vi "Get All CEID Data.vi"(8 "error in (no error)":errorcluster) -> (0 "error out":errorcluster, 3 "CEID Data":T1[](array[typedef]))   [LabVIEW 2020, in "SECS Communication.lvlib" / "SECS Data Class.lvclass"]
uses:
  SECS Data Class.lvclass
  CEID Data.ctl
  SECS Data Class.lvclass/SECS Data Class.ctl
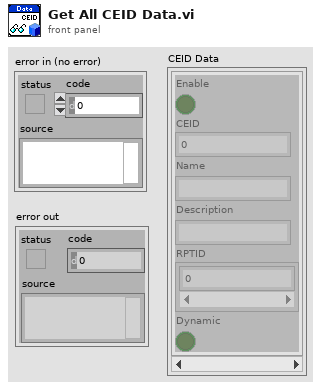
[diagram p1: front panel]
types:
  T1 = typedef "SECS Communication.lvlib/SECS Data Class.lvclass/CEID Data.ctl" = cluster{"Enable":bool, "CEID":u32, "Name":string, "Description":string, "RPTID":u32[], "Dynamic":bool}
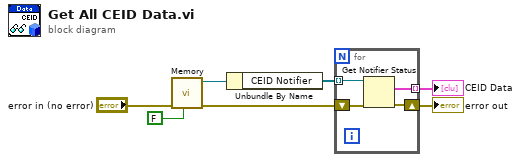
[diagram p0: block diagram]
diagram:
  n1 = call "Memory.vi"("Put"=FALSE, "error in (no error)"="error in (no error)") -> ("error out"=w4:errorcluster, "SECS Data Class out"=w5:refnum<class "SECS Data Class.lvclass">)  [unwired: 8 in]
  n2 = Unbundle By Name(w5) -> ("CEID Notifier"=w3:refnum<notifier>[])
  n3 = for {
    shift-right: [w9] -> w1
    shift-left: w4 -> [w10]
    tunnel: w3 -> [w11] mode=indexing
    tunnel: [w8] -> w2 mode=indexing
    n4 = Get Notifier Status(notifier=w11, error in (no error)=w10) -> (current notification=w8:T1, error out=w9:errorcluster)  [unwired: 3 out]
  }
  "error out" <- w1
  "CEID Data" <- w2
